vi "String_conc.vi"() -> ()   [LabVIEW 2019]
panel:
  out "Result":string
  in  "String 2":string="Dudharejiya"
  in  "String":string="Ankit"
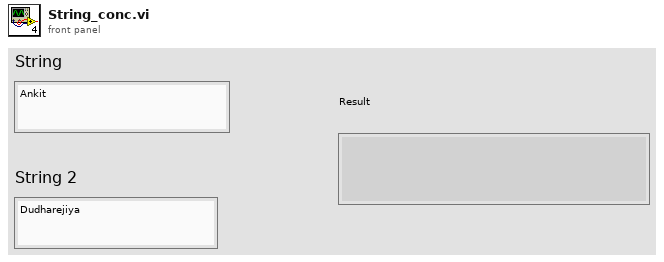
[diagram p1: front panel]
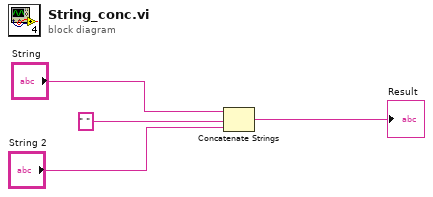
[diagram p0: block diagram]
diagram:
  n1 = Concatenate Strings("String", " ", "String 2") -> (→"Result":string)
